vi "convert_to_unit.vi"(7 "unit_dictionary":variant, 8 "error in (no error)":errorcluster, 9 "unit_to":string, 10 "unit_from":string, 11 "value in":dbl) -> (0 "error out":errorcluster, 3 "value out":dbl)   [LabVIEW 2015, in "lv-unit-conversion.lvlib"]
uses:
  lv-unit-conversion.lvlib
  _controls/error.ctl
  _controls/unit.ctl
panel:
  out "unit out":string
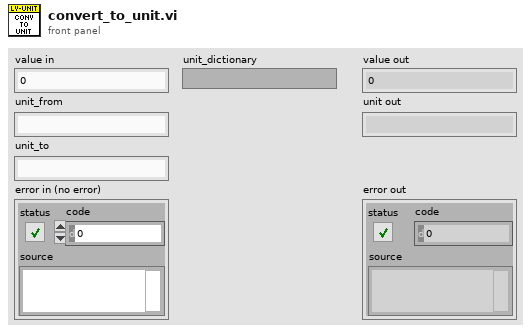
[diagram p1: front panel]
types:
  T1 = typedef "lv-unit-conversion.lvlib/error.ctl" = enum16{"<lv-unit-conversion_error>", "unit_not_found", "xml_parser", "<null>"}
  T2 = typedef "lv-unit-conversion.lvlib/unit.ctl" = cluster{"symbol":string, "name":string, "dimension":string, "is_si_unit":bool, "category":string, "base_unit":string, "conversion_reference":string, "is_exact":bool, "a":dbl, "b":dbl, "c":dbl, "d":dbl, "underlying_def":string, "description":string}
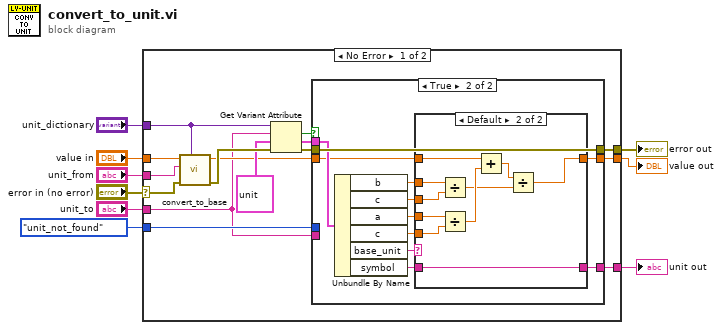
[diagram p0: block diagram]
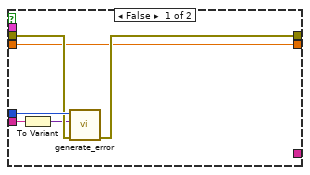
[diagram p2: hidden frame]
diagram:
  n1 = case shown="No Error" "error in (no error)" {
    selector: "error in (no error)" -> [w11 w54]
    tunnel: "unit_dictionary" -> [w15 _]
    tunnel: "value in" -> [w14 _]
    tunnel: [w22 _] -> w6
    tunnel: [w21 _] -> w5
    tunnel: [w18 w54] -> w4
    tunnel: error."unit_not_found" ("error") -> [w17 _]
    tunnel: "unit_from" -> [w12 _]
    tunnel: "unit_to" -> [w10 _]
    frame No Error {
      n2 = call "convert_to_base.vi"("unit_set"=w15, "error in (no error)"=w11, "unit in"=w12, "value in"=w14) -> ("error out"=w24:errorcluster, "value out"=w13:dbl)  [unwired: 6 in]
      n3 = Get Variant Attribute(Variant=w15, name=w10, default value (empty Variant)=T2 {"symbol"="", "name"="", "dimension"="", "is_si_unit"=FALSE, "category"="", "base_unit"="", "conversion_reference"="", "is_exact"=FALSE, "a"=0.0, "b"=0.0, "c"=0.0, "d"=0.0, "underlying_def"="", "description"=""} ("unit_set"), error in=w24) -> (found=w20:bool, value=w23:T2, error out=w19:errorcluster)  [unwired: 1 out]
      n4 = case shown="True" w20 {
        tunnel: w23 -> [_ w40]
        tunnel: w13 -> [w25 w39]
        tunnel: [w25 w38] -> w22
        tunnel: [_ w31] -> w21
        tunnel: w19 -> [w29 w41]
        tunnel: [w28 w41] -> w18
        tunnel: w17 -> [w30 _]
        tunnel: w10 -> [w27 _]
        frame False {
          n5 = To Variant(anything=w27) -> (Variant=w26:variant)
          n6 = call "generate_error.vi"("error in (no error)"=w29, "data"=w26, "error"=w30) -> ("error out"=w28:errorcluster)  [unwired: 8 in]
        }
        frame True {
          n7 = Unbundle By Name(w40) -> ("b"=w37:dbl, "c"=w36:dbl, "a"=w35:dbl, "c"=w34:dbl, "base_unit"=w33:string, "symbol"=w32:string)
          n8 = case shown="Default" w33 {
            tunnel: w39 -> [w43 w48]
            tunnel: [w43 w44] -> w38
            tunnel: w37 -> [_ w53]
            tunnel: w36 -> [_ w52]
            tunnel: w35 -> [_ w51]
            tunnel: w34 -> [_ w50]
            tunnel: w32 -> [w42 w49]
            tunnel: [w42 w49] -> w31
            frame "" {
            }
            frame Default {
              n9 = Divide(x=w53, y=w52) -> (x/y=w45:dbl)
              n10 = Divide(x=w51, y=w50) -> (x/y=w47:dbl)
              n11 = Add(x=w48, y=w47) -> (x+y=w46:dbl)
              n12 = Divide(x=w46, y=w45) -> (x/y=w44:dbl)
            }
          }
        }
      }
    }
    frame Error {
    }
  }
  "value out" <- w6
  "error out" <- w4
  "unit out" <- w5
